vi "UUT Result Dialog.vi"(10 "Select Dialog":T1(ring)=enum."Failed") -> ()   [LabVIEW 2010]
uses:
  _TypeDefs/OK Button_TouchScreen.ctl
panel:
  out "Message":string
  in  "OK":T2
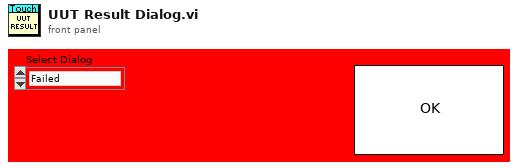
[diagram p1: front panel]
types:
  T1 = enum16{"Passed", "Failed", "Error", "Terminated"}
  T2 = typedef "OK Button_TouchScreen.ctl" = bool
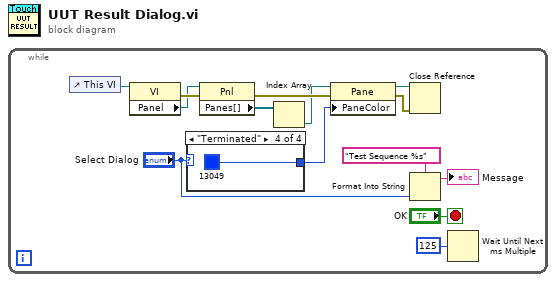
[diagram p0: block diagram]
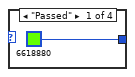
[diagram p2: hidden frame]
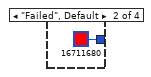
[diagram p3: hidden frame]
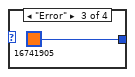
[diagram p4: hidden frame]
diagram:
  n1 = while {
    stop <- "OK" stop-if-true
    n2 = control-ref of="This VI"() -> (w1:refnum<vi>)
    n3 = property class="VI"(reference=w1) -> (error out=w8:errorcluster, "Panel"=w7:refnum<vi>)  [unwired: 1 in, 1 out]
    n4 = case shown="\"Terminated\"" "Select Dialog" {
      tunnel: [u32 6618880 u32 16711680 u32 16741905 u32 13049] -> w2
      frame "Passed" {
      }
      frame "Failed", Default {
      }
      frame "Error" {
      }
      frame "Terminated" {
      }
    }
    n5 = property class="Pnl"(reference=w7, error in=w8) -> (error out=w6:errorcluster, "Panes[]"=w9:refnum<vi>[])  [unwired: 1 out]
    n6 = Index Array(array=w9) -> (element=w5:refnum<vi>)  [unwired: 1 in]
    n7 = property class="Pane"(reference=w5, error in=w6, "PaneColor"=w2) -> (reference out=w4:refnum<vi>, error out=w3:errorcluster)
    n8 = Close Reference(reference=w4, error in (no error)=w3) -> ()  [unwired: 1 out]
    n9 = Format Into String(format string="Test Sequence %s" ("Message"), "Select Dialog") -> (resulting string=→"Message":string)  [unwired: 2 in, 1 out]
    n10 = Wait Until Next ms Multiple(millisecond multiple=u32 125) -> ()  [unwired: 1 out]
  }
